vi "Write Run Url File.vi"(8 "Sift Client in":refnum<class "Sift Client.lvclass">, 10 "TDMS Filepath":path, 11 "Run URL":string) -> ()   [LabVIEW 2024, in "Sift TDMS Uploader.lvlib" / "Sift TDMS Uploader.lvclass"]
uses:
  Sift TDMS Uploader.lvclass
  <vilib>/Sift/Sift/Sift API/Sift Client.lvclass
  <vilib>/Utility/config.llb/Write Key (String).vi
  Sift TDMS Uploader.lvclass/Sift TDMS Uploader.ctl
  <vilib>/Utility/config.llb/NI_LVConfig.lvlib
panel:
  out "error out":errorcluster
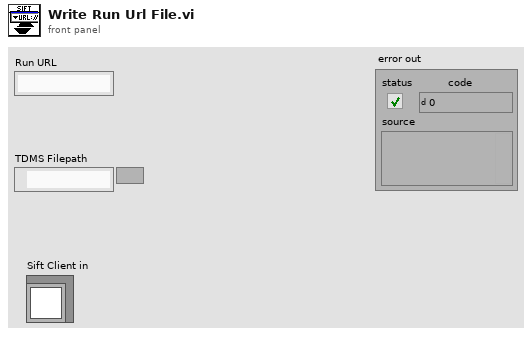
[diagram p1: front panel]
types:
  T1 = typedef "NI_LVConfig.lvlib/Config Data RefNum.ctl" = refnum<k1>
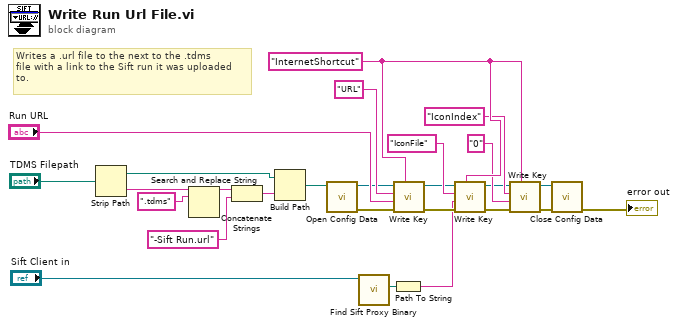
[diagram p0: block diagram]
diagram:
  w24 = "InternetShortcut"
  # "Writes a .url file to the next to the .tdms\nfile with a link to the Sift run it was uploaded\nto."
  n1 = Strip Path(path="TDMS Filepath") -> (stripped path=w6:path, name=w8:string)
  n2 = Search and Replace String(input string=w8, search string=".tdms") -> (result string=w9:string)  [unwired: 6 in, 3 out]
  n3 = Concatenate Strings(w9, "-Sift Run.url") -> (w11:string)
  n4 = Build Path(base path=w6, name or relative path=w11) -> (appended path=w12:path)
  n5 = call <vilib>:"Open Config Data.vi"("configuration file path"=w12) -> ("error out"=w18:errorcluster, "refnum"=w13:T1)  [unwired: 8 in, 1 out]
  n6 = call-dynamic "Find Sift Proxy Binary.vi"("Sift Client in"="Sift Client in") -> ("Path"=w1:path)  [unwired: 7 in, 3 out]
  n7 = Path To String(path=w1) -> (string=w2:string)
  n8 = call-poly <vilib>:"Write Key.vi"("section"=w24, "error in (no error)"=w18, "value"="Run URL", "key"="URL", "refnum"=w13) -> ("error out"=w19:errorcluster, "refnum out"=w15:T1)  [unwired: 4 in, 1 out]
  n9 = call-poly <vilib>:"Write Key.vi"("section"=w24, "error in (no error)"=w19, "value"=w2, "key"="IconFile", "refnum"=w15) -> ("error out"=w20:errorcluster, "refnum out"=w21:T1)  [unwired: 4 in, 1 out]
  n10 = call-poly <vilib>:"Write Key.vi"("section"=w24, "error in (no error)"=w20, "value"="0", "key"="IconIndex", "refnum"=w21) -> ("error out"=w26:errorcluster, "refnum out"=w25:T1)  [unwired: 4 in, 1 out]
  n11 = call <vilib>:"Close Config Data.vi"("error in (no error)"=w26, "refnum"=w25) -> ("error out"=→"error out":errorcluster)  [unwired: 8 in, 1 out]
